vi "Write Glue Speed.vi"(8 "error in (no error)":errorcluster, 10 "Glue Speed":i32, 11 "Crosshair Dispense in":refnum<class "Crosshair Dispense.lvclass">) -> (0 "error out":errorcluster, 3 "Crosshair Dispense out":refnum<class "Crosshair Dispense.lvclass">)   [LabVIEW 2019, in "Crosshair Dispense.lvclass"]
uses:
  Crosshair Dispense.lvclass
  Crosshair Dispense.lvclass/Crosshair Dispense.ctl
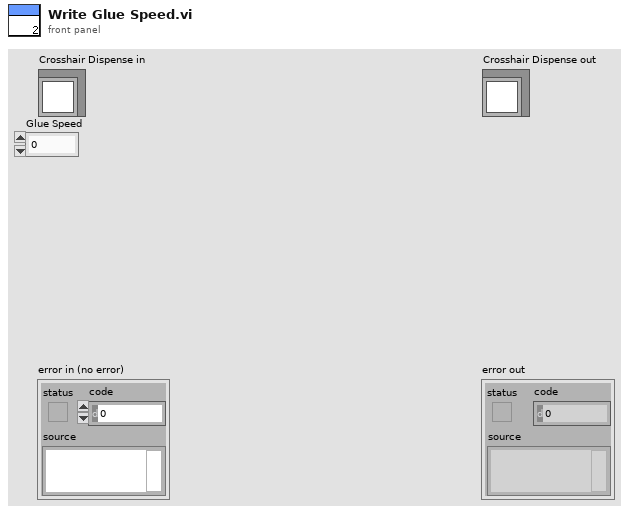
[diagram p1: front panel]
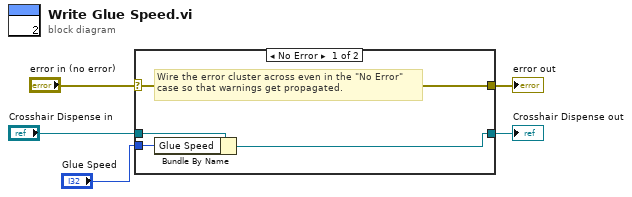
[diagram p0: block diagram]
diagram:
  n1 = case shown="No Error" "error in (no error)" {
    selector: "error in (no error)" -> [w9 w11]
    tunnel: [w9 w11] -> w4
    tunnel: [w6 w10] -> w2
    tunnel: "Crosshair Dispense in" -> [w8 w10]
    tunnel: "Glue Speed" -> [w7 _]
    frame No Error {
      # "Wire the error cluster across even in the \"No Error\"\ncase so that warnings get propagated."
      n2 = Bundle By Name(cluster=w8, "Glue Speed"=w7) -> (w6:refnum<class "Crosshair Dispense.lvclass">)
    }
    frame Error {
    }
  }
  "error out" <- w4
  "Crosshair Dispense out" <- w2
